vi "OSA_example_option.vi"() -> ()   [LabVIEW 2010]
doc: "PD TIA gain setting example showing how the autogain works (at different modes) and the benefit of manual gain setting."
uses:
  _OSA_class/OSA.lvclass
  _OSA_class/typeDef/resolution.ctl
  _OSA_class/typeDef/sensitivityMode.ctl
panel:
  in  "sensitivity":T1=enum."high"
  in  "gain_idx":u16 max=50
  in  "gain auto":bool
  in  "stop":bool
  out "Intensity Graph Interferogram":i32[][](graph)
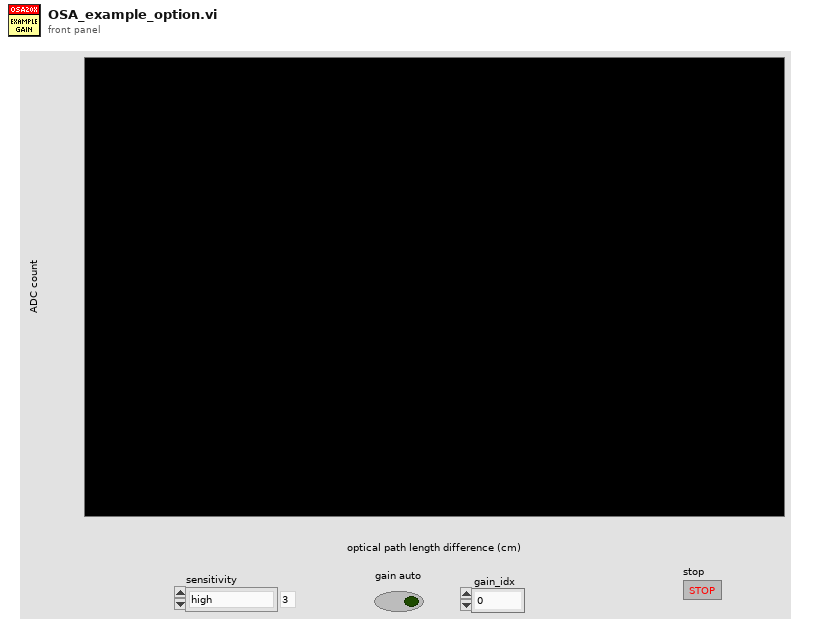
[diagram p1: front panel]
types:
  T1 = typedef "OSA.lvclass/sensitivityMode.ctl" = enum16{"low", "low medium", "high medium", "high"}
  T2 = typedef "OSA.lvclass/resolution.ctl" = enum16{"low", "high"}
  T3 = typedef "OSA.lvclass/acq_dataType.ctl" = enum16{"none", "interferogram", "spectrum"}
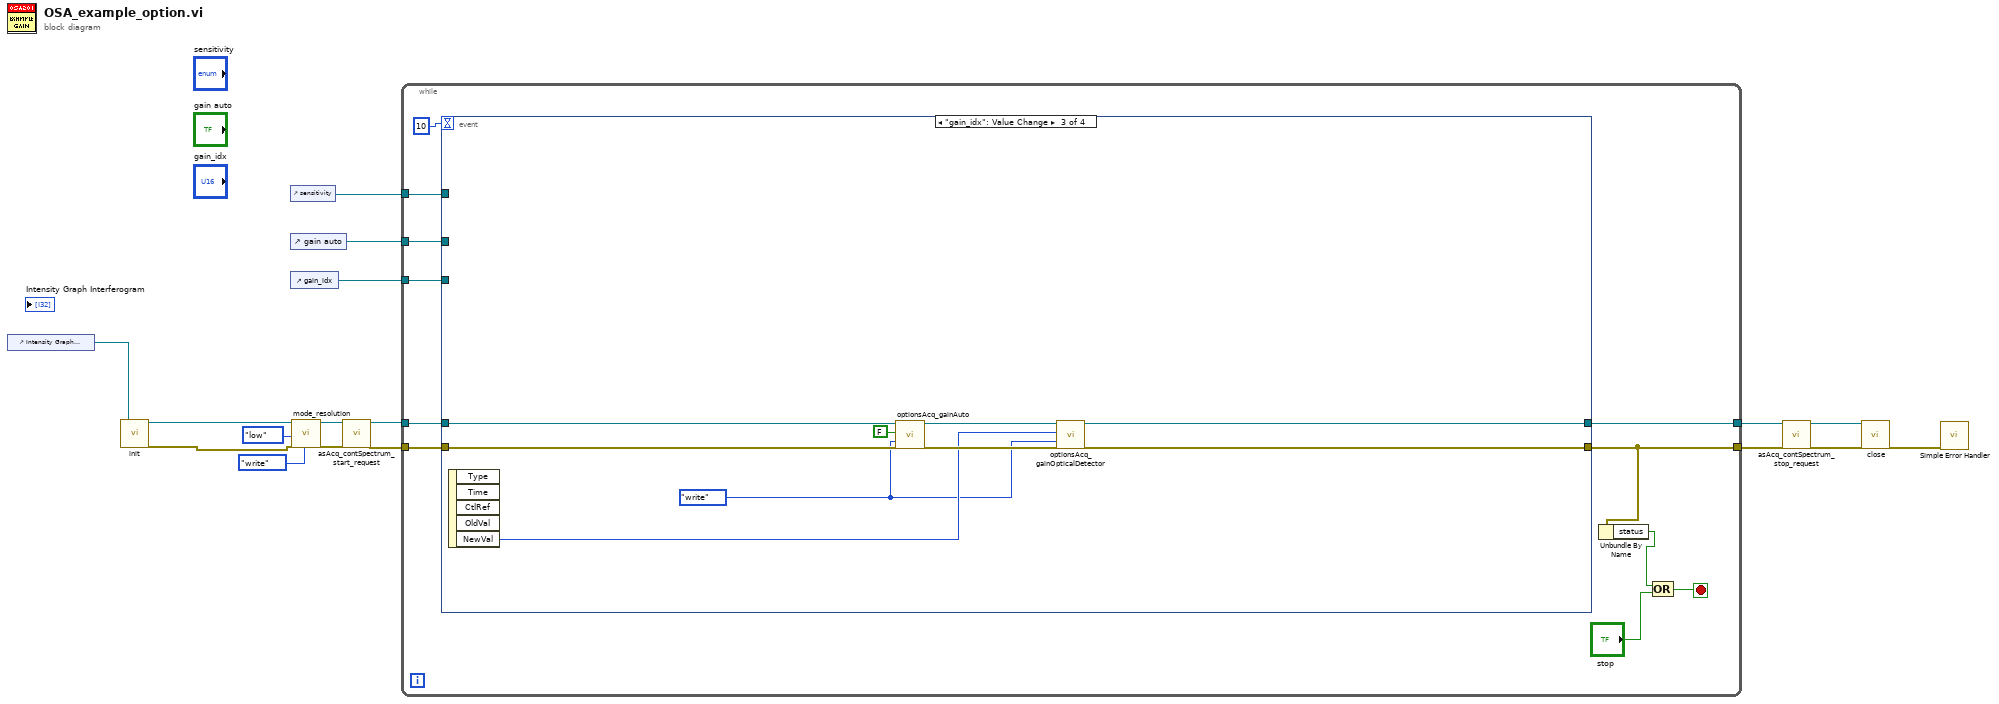
[diagram p0: block diagram]
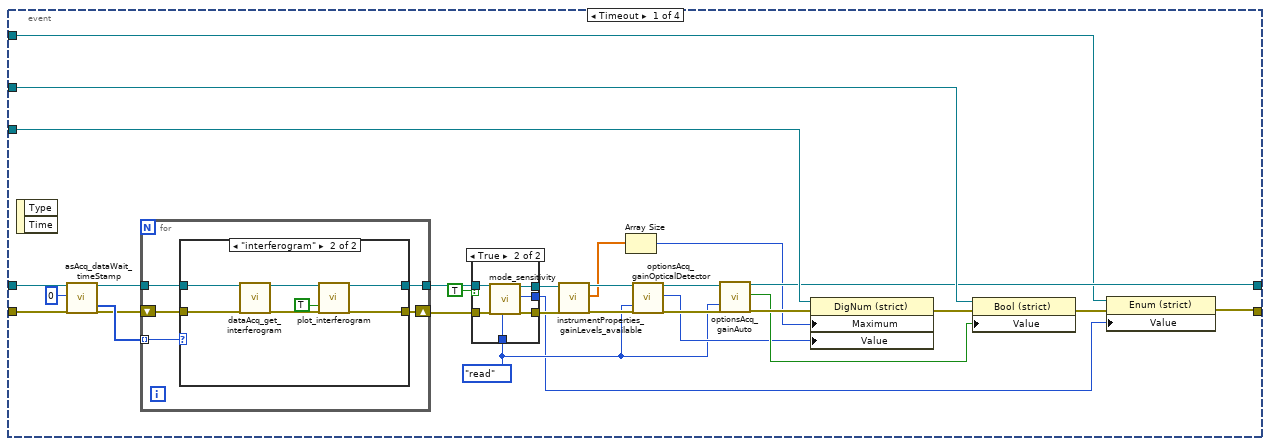
[diagram p2: hidden frame]
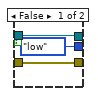
[diagram p3: hidden frame]
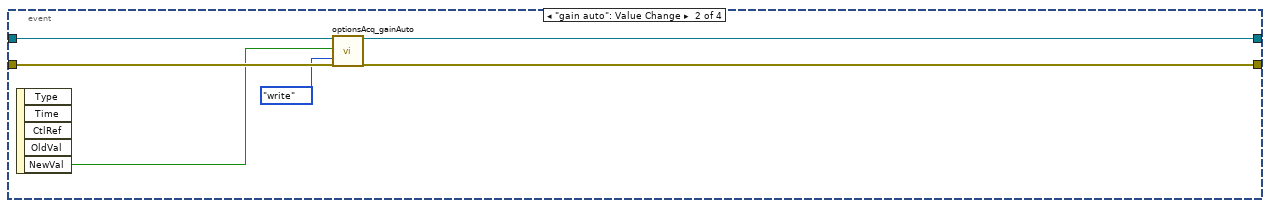
[diagram p5: hidden frame]
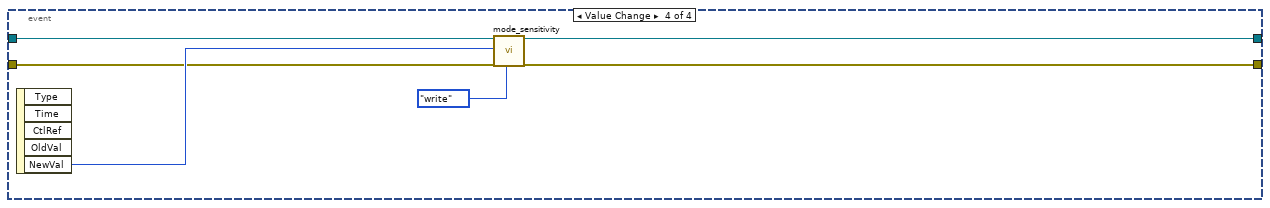
[diagram p6: hidden frame]
diagram:
  n1 = control-ref of="Intensity Graph Interferogram"() -> (w17:refnum<vi>)
  n2 = call "init.vi"("Graph Intrfrgrm"=w17) -> ("duplicate reference"=w2:refnum<class "OSA.lvclass">, "error out"=w1:errorcluster)  [unwired: 14 in, 3 out]
  n3 = control-ref of="gain auto"() -> (w12:refnum<vi>)
  n4 = control-ref of="gain_idx"() -> (w11:refnum<vi>)
  n5 = control-ref of="sensitivity"() -> (w8:refnum<vi>)
  n6 = call "mode_resolution.vi"("reference"=w2, "resolution"=resolution."low", "error in (no error)"=w1, "read/write"=enum16{"read", "write"}."write") -> ("duplicate reference"=w3:refnum<class "OSA.lvclass">, "error out"=w6:errorcluster)  [unwired: 12 in, 2 out]
  n7 = call "asAcq_contSpectrum_start_request.vi"("reference"=w3, "error in (no error)"=w6) -> ("duplicate reference"=w4:refnum<class "OSA.lvclass">, "error out"=w5:errorcluster)  [unwired: 16 in]
  n8 = while {
    tunnel: w4 -> [w28]
    tunnel: w5 -> [w27]
    tunnel: [w19] -> w16
    tunnel: [w26] -> w15
    tunnel: w12 -> [w24]
    tunnel: w11 -> [w23]
    tunnel: w8 -> [w20]
    stop <- w22 stop-if-true
    n9 = event shown="[2] \"gain_idx\": Value Change" {
      selector: _ -> [_ _ _ _]
      dyn-events: _ -> [_ _ _ _]
      timeout: 10 -> [_ _ _ _]
      tunnel: w28 -> [w57 w83 w92 w99]
      tunnel: w27 -> [w55 w86 w93 w98]
      tunnel: [w31 w85 w94 w97] -> w19
      tunnel: [w45 w82 w95 w96] -> w26
      tunnel: w24 -> [w47 _ _ _]
      tunnel: w23 -> [w49 _ _ _]
      tunnel: w20 -> [w32 _ _ _]
      event Timeout {
        w34 = enum16{"read", "write"}."read" ("readWrite")
        n10 = event-data() -> ()  [unwired: 1 in, 2 out]
        n11 = call "asAcq_dataWait_timeStamp.vi"("reference"=w57, "ms wait"=0, "error in (no error)"=w55) -> ("duplicate reference"=w56:refnum<class "OSA.lvclass">, "dataType"=w54:T3[], "error out"=w53:errorcluster)  [unwired: 14 in]
        n12 = for {
          tunnel: w56 -> [w71]
          tunnel: [w70] -> w36
          tunnel: w54 -> [w69] mode=indexing
          shift-right: [w67] -> w38
          shift-left: w53 -> [w68]
          n13 = case shown="\"interferogram\"" w69 {
            tunnel: w71 -> [w72 w80]
            tunnel: w68 -> [w73 w78]
            tunnel: [w73 w76] -> w67
            tunnel: [w72 w75] -> w70
            frame "none", Default {
            }
            frame "interferogram" {
              n14 = call-dynamic "dataAcq_get_interferogram.vi"("reference"=w80, "error in (no error)"=w78) -> ("duplicate reference"=w79:refnum<class "OSA.lvclass">, "error out"=w77:errorcluster)  [unwired: 16 in]
              n15 = call "plot_interferogram.vi"("reference"=w79, "autoScale Y"=TRUE, "error in (no error)"=w77) -> ("duplicate reference"=w75:refnum<class "OSA.lvclass">, "error out"=w76:errorcluster)  [unwired: 15 in]
            }
          }
        }
        n16 = case shown="True" TRUE {
          tunnel: w38 -> [w59 w66]
          tunnel: [w59 w65] -> w37
          tunnel: w36 -> [w60 w64]
          tunnel: [w60 w63] -> w35
          tunnel: w34 -> [_ w62]
          tunnel: [sensitivityMode."low" ("sensitivity out") w61] -> w30
          frame False {
          }
          frame True {
            n17 = call "mode_sensitivity.vi"("reference"=w64, "error in (no error)"=w66, "read/write"=w62) -> ("duplicate reference"=w63:refnum<class "OSA.lvclass">, "sensitivity out"=w61:T1, "error out"=w65:errorcluster)  [unwired: 14 in]
          }
        }
        n18 = call "instrumentProperties_gainLevels_available.vi"("reference"=w35, "error in (no error)"=w37) -> ("duplicate reference"=w42:refnum<class "OSA.lvclass">, "gainLevels out"=w41:dbl[], "error out"=w43:errorcluster)  [unwired: 15 in]
        n19 = Array Size(array=w41) -> (size(s)=w39:i32)
        n20 = call-dynamic "optionsAcq_gainOpticalDetector.vi"("reference"=w42, "readWrite"=w34, "error in (no error)"=w43) -> ("duplicate reference"=w51:refnum<class "OSA.lvclass">, "gain_idx  out"=w40:u16, "error out"=w50:errorcluster)  [unwired: 12 in, 2 out]
        n21 = call-dynamic "optionsAcq_gainAuto.vi"("reference"=w51, "readWrite"=w34, "error in (no error)"=w50) -> ("duplicate reference"=w45:refnum<class "OSA.lvclass">, "auto out"=w44:bool, "error out"=w48:errorcluster)  [unwired: 13 in, 1 out]
        n22 = property class="DigNum (strict)"(reference=w49, error in=w48, "Maximum"=w39, "Value"=w40) -> (error out=w46:errorcluster)  [unwired: 1 out]
        n23 = property class="Bool (strict)"(reference=w47, error in=w46, "Value"=w44) -> (error out=w33:errorcluster)  [unwired: 1 out]
        n24 = property class="Enum (strict)"(reference=w32, error in=w33, "Value"=w30) -> (error out=w31:errorcluster)  [unwired: 1 out]
      }
      event "gain auto": Value Change {
        n25 = event-data() -> ("NewVal"=w84:bool)  [unwired: 1 in, 4 out]
        n26 = call-dynamic "optionsAcq_gainAuto.vi"("reference"=w83, "auto"=w84, "readWrite"=enum16{"read", "write"}."write", "error in (no error)"=w86) -> ("duplicate reference"=w82:refnum<class "OSA.lvclass">, "error out"=w85:errorcluster)  [unwired: 12 in, 2 out]
      }
      event "gain_idx": Value Change {
        w87 = enum16{"read", "write"}."write" ("readWrite")
        n27 = event-data() -> ("NewVal"=w89:u16)  [unwired: 1 in, 4 out]
        n28 = call-dynamic "optionsAcq_gainAuto.vi"("reference"=w92, "auto"=FALSE, "readWrite"=w87, "error in (no error)"=w93) -> ("duplicate reference"=w91:refnum<class "OSA.lvclass">, "error out"=w90:errorcluster)  [unwired: 12 in, 2 out]
        n29 = call-dynamic "optionsAcq_gainOpticalDetector.vi"("reference"=w91, "gain_idx"=w89, "readWrite"=w87, "error in (no error)"=w90) -> ("duplicate reference"=w95:refnum<class "OSA.lvclass">, "error out"=w94:errorcluster)  [unwired: 11 in, 3 out]
      }
      event Value Change {
        n30 = event-data() -> ("NewVal"=w100:T1)  [unwired: 1 in, 4 out]
        n31 = call "mode_sensitivity.vi"("reference"=w99, "sensitivity"=w100, "error in (no error)"=w98, "read/write"=enum16{"read", "write"}."write") -> ("duplicate reference"=w96:refnum<class "OSA.lvclass">, "error out"=w97:errorcluster)  [unwired: 13 in, 1 out]
      }
    }
    n32 = Unbundle By Name(w19) -> ("status"=w18:bool)
    n33 = Compound Arithmetic op=OR(w18, "stop") -> (w22:bool)
  }
  n34 = call "asAcq_contSpectrum_stop_request.vi"("reference"=w15, "error in (no error)"=w16) -> ("duplicate reference"=w13:refnum<class "OSA.lvclass">, "error out"=w14:errorcluster)  [unwired: 16 in]
  n35 = call "close.vi"("reference"=w13, "error in (no error)"=w14) -> ("error out"=w10:errorcluster)  [unwired: 17 in]
  n36 = call <vilib>:"Simple Error Handler.vi"("error in (no error)"=w10) -> ()  [unwired: 4 in, 5 out]
